vi "Fishing Continuous OCR wit Max Likelihood P Stimuli.vi"() -> ()   [LabVIEW 2019]
doc: "This VI captures the region of the screen and displays it on the front panel continuously.\nCan be used to develop remote desktop applications."
uses:
  System.Drawing
  <vilib>/wsapi/NI_WebServices.lvlib
  <vilib>/Utility/miscctls.llb/LVBoundsTypeDef.ctl
  <vilib>/Utility/inputDevices.llb/closeMouse.vi
  <vilib>/Instr/_visa.llb/VISA Configure Serial Port (Instr).vi
  <vilib>/Utility/inputDevices.llb/mouseAcquire.vi
panel:
  in  "P Trig":bool
  out "P Command":string
  in  "P Stimuli":bool
  out "Length":i32
  out "Array Reset":bool
  out "TXB":bool
  out "Scan Cycle":dbl
  out "read buffer":string
  out "Max Likelihood Output":string
  out "Max Index":i32
  in  "Manual Reset Array":bool
  out "Input Likelihood":dbl[](array[numeric])
  out "Possible Inputs":string[](array[string])
  out "Init Error":errorcluster
  out "Tx":string
  out "Return Count":u32
  out "COM Status":bool
  in  "MC COM Port":refnum<visa-resource-name>="COM5"
  out "Processed Image":T1(plugin-control)
  out "Filtered String Output":string
  in  "Delay (ms)":i32=100
  in  "Error In":errorcluster
  out "Mouse y":dbl
  out "Mouse x":dbl
  in  "Height (px)":i32=100
  in  "Width (px)":i32=600
  out "Screen Capture":picture
  in  "stop":bool
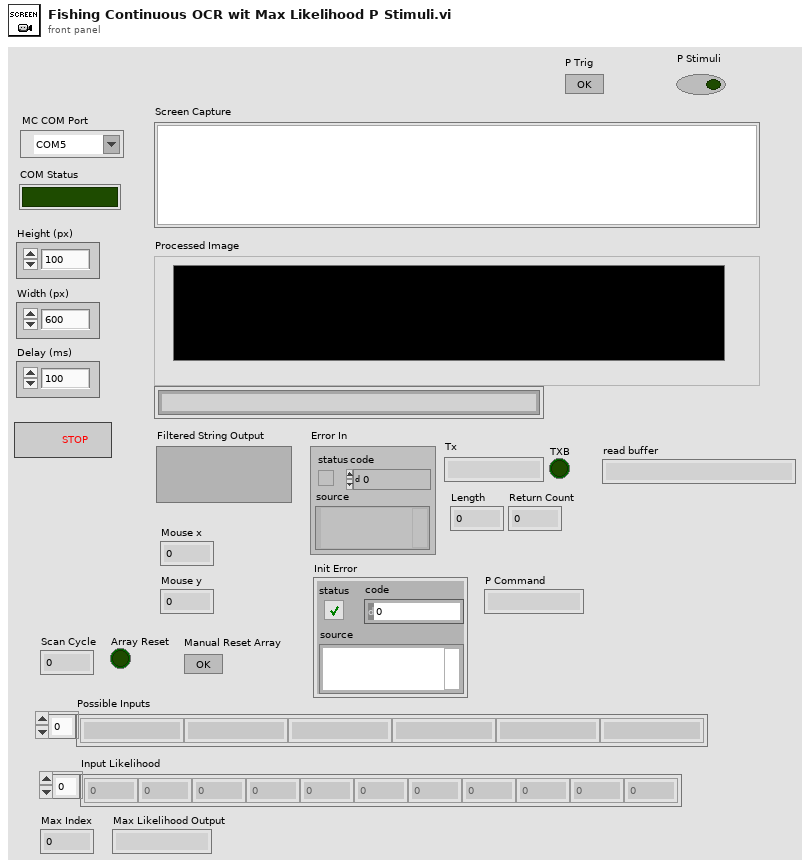
[diagram p1: front panel]
types:
  T1 = typedef "IMAQ Image.ctl" = refnum<image>
  T2 = typedef "LVBoundsTypeDef.ctl" = cluster{"Width":u32, "Height":u32}
  T3 = typedef "Image Type" = u32
  T4 = cluster{"Horizontal":i32, "Vertical":i32, "Scrolling":i32}
  T5 = typedef "imagedata.ctl" = cluster{"image type":i32, "image depth":i32, "image":u8[], "mask":u8[], "colors":u32[], "Rectangle":cluster{"left":i16, "top":i16, "right":i16, "bottom":i16}}
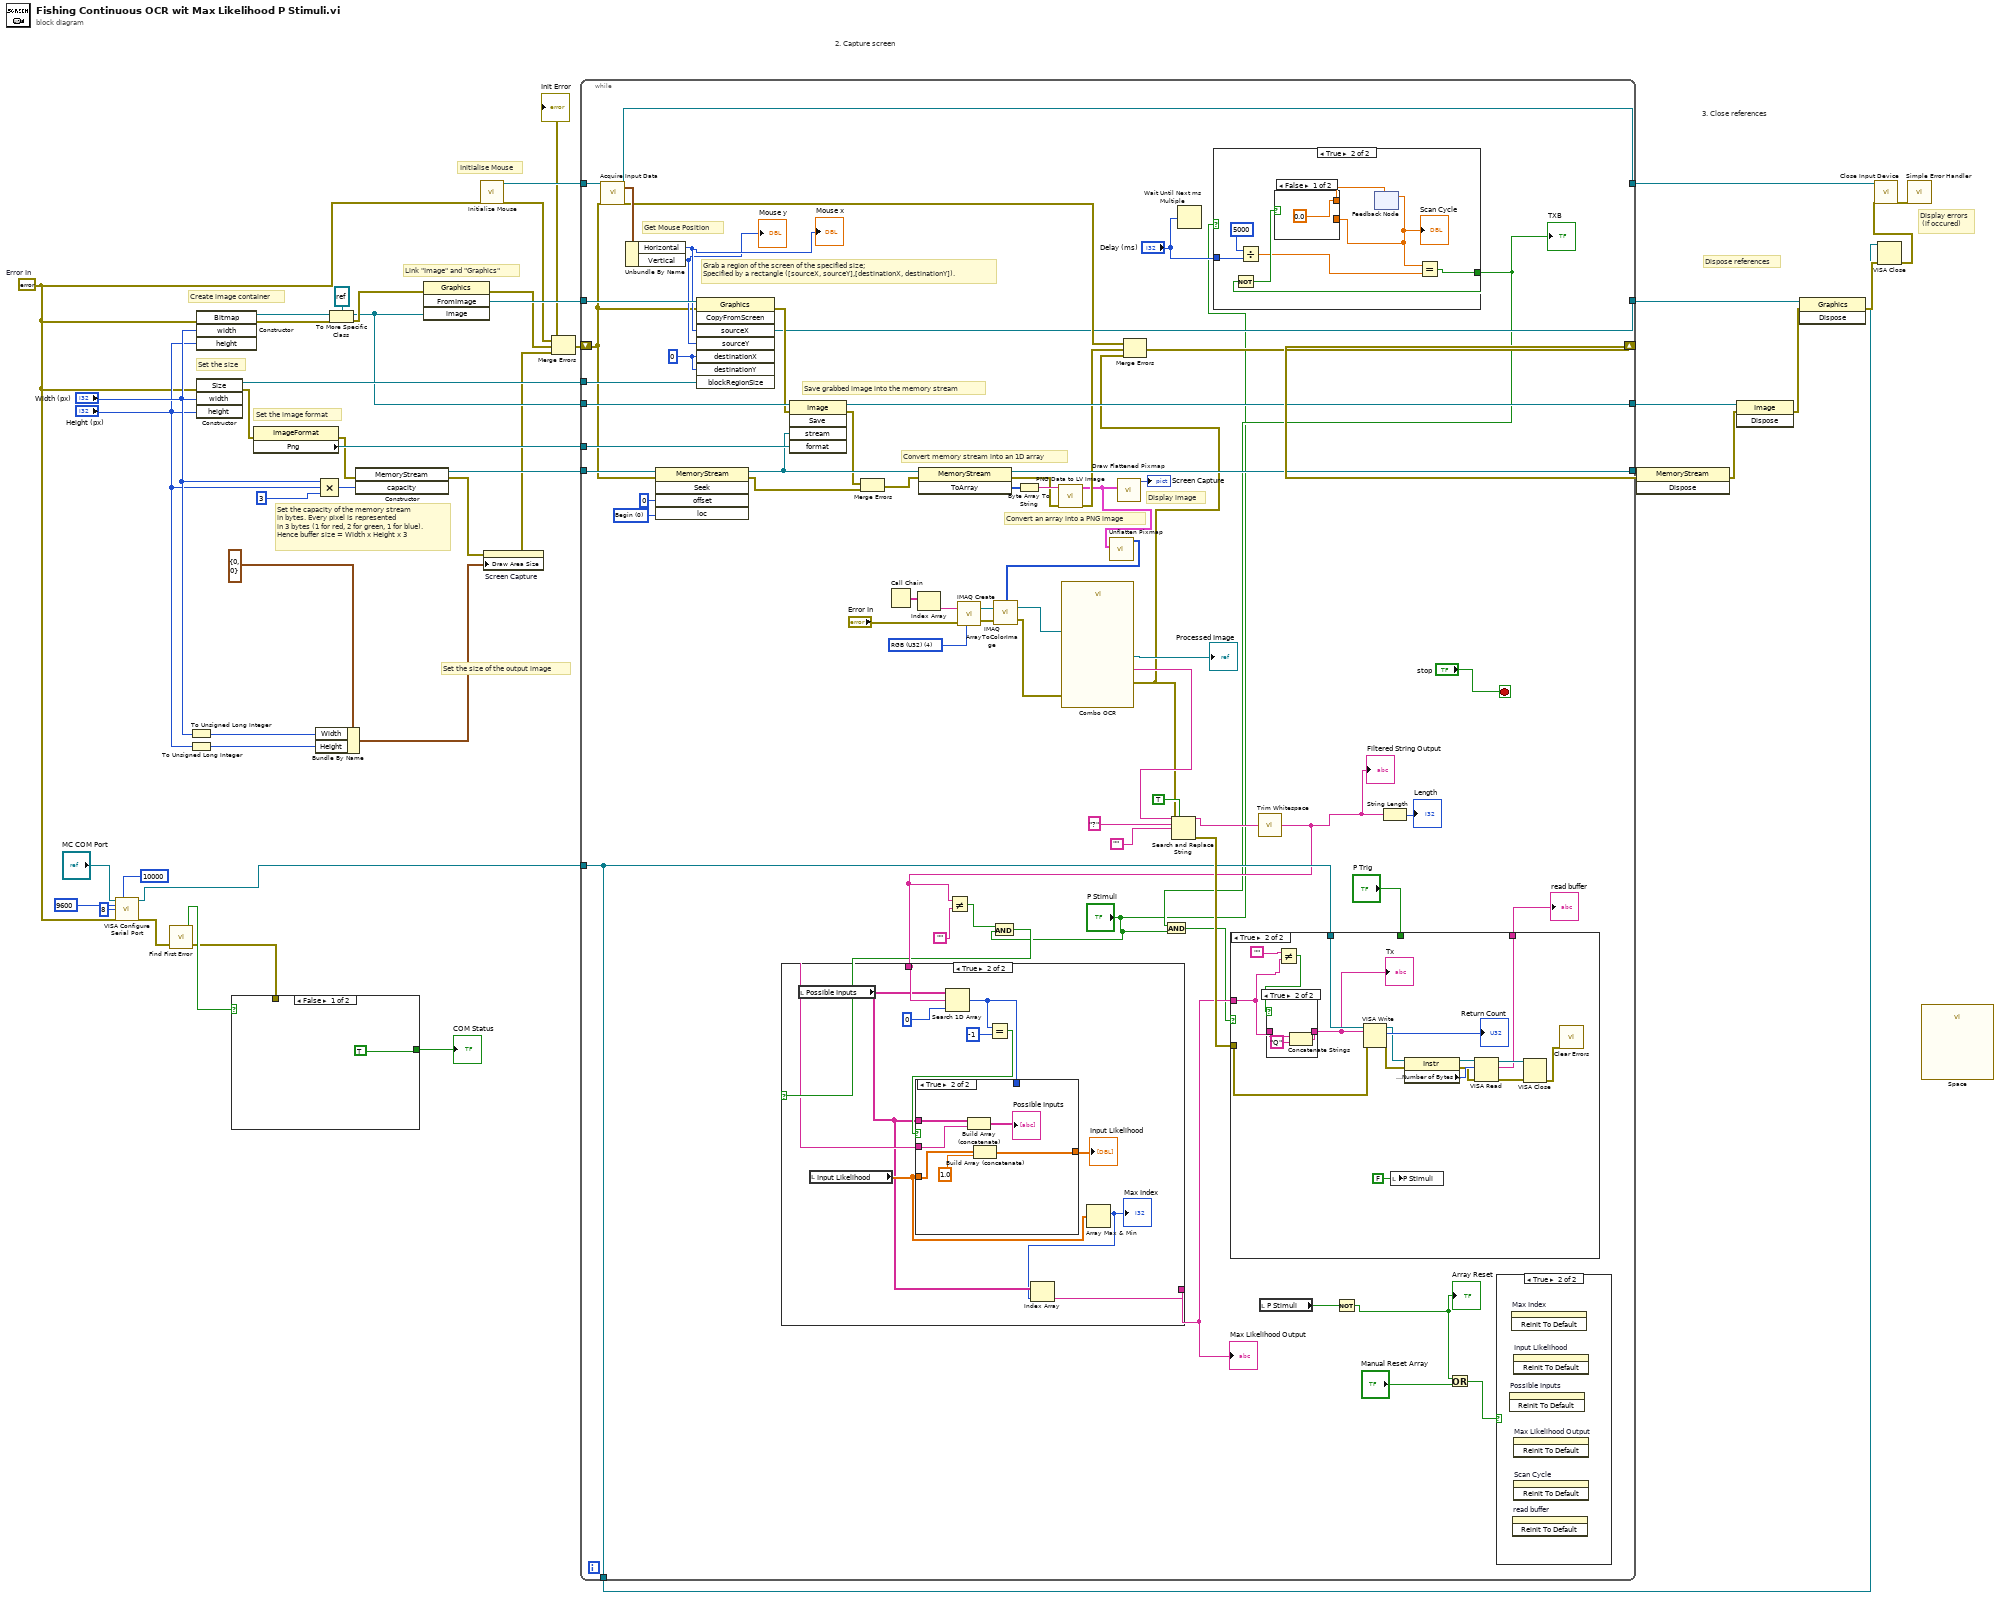
[diagram p0: block diagram]
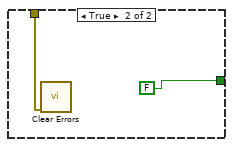
[diagram p2: hidden frame]
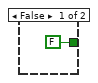
[diagram p3: hidden frame]
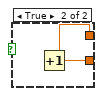
[diagram p4: hidden frame]
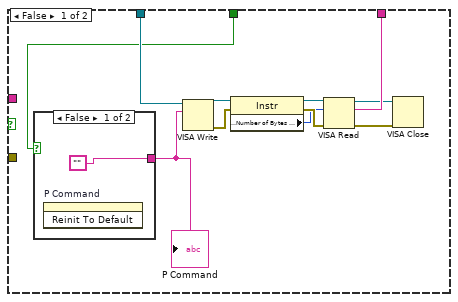
[diagram p5: hidden frame]
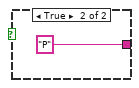
[diagram p6: hidden frame]
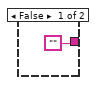
[diagram p7: hidden frame]
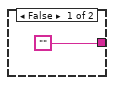
[diagram p8: hidden frame]
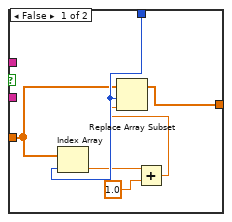
[diagram p9: hidden frame]
diagram:
  w12 = errorcluster {"status"=FALSE, "code"=0, "source"=""}  # Error In
  # "Link \"Image\" and \"Graphics\""
  # "Set the size"
  # "Create image container"
  # "3. Close references"
  # "2. Capture screen"
  # "Display errors\n (if occured)"
  # "Dispose references"
  # "Set the image format"
  # "Set the size of the output image"
  # "Set the capacity of the memory stream\nin bytes. Every pixel is represented\nin 3 bytes (1 for red, 2 for green, 1 for blue).\nHence buffer size = Width x Height x 3"
  # "Initialise Mouse"
  n1 = call-poly "VISA Configure Serial Port"("VISA resource name"="MC COM Port", "timeout (10sec)"=u32 10000, "baud rate (9600)"=u32 9600, "data bits (8)"=u16 8, "error in (no error)"=w12) -> ("VISA resource name out"=w1:refnum<visa-resource-name>, "error out"=w11:errorcluster)  [unwired: 9 in]
  n2 = call <vilib>:"Find First Error.vi"("error in (no error)"=w11) -> ("error out"=w8:errorcluster, "error?"=w10:bool)  [unwired: 3 in]
  n3 = To Unsigned Long Integer(number="Width (px)") -> (unsigned 32bit integer=w20:u32)
  n4 = To Unsigned Long Integer(number="Height (px)") -> (unsigned 32bit integer=w18:u32)
  n5 = constructor class="Bitmap"(error in=w12, "width"="Width (px)", "height"="Height (px)") -> (reference out=w40:refnum<k24>, error out=w43:errorcluster)  [unwired: 2 in, 3 out]
  n6 = constructor class="Size"(error in=w12, "width"="Width (px)", "height"="Height (px)") -> (reference out=w38:refnum<k24>, error out=w29:errorcluster)  [unwired: 2 in, 3 out]
  n7 = case shown="False" w10 {
    tunnel: [TRUE FALSE] -> w9
    tunnel: w8 -> [_ w48]
    frame False {
    }
    frame True {
      n8 = call <vilib>:"Clear Errors.vi"("error in (no error)"=w48) -> ()  [unwired: 5 in, 2 out]
    }
  }
  "COM Status" <- w9
  n9 = property class="ImageFormat"(error in=w29) -> (error out=w28:errorcluster, "Png"=w37:refnum<k24>)  [unwired: 1 in, 1 out]
  n10 = Bundle By Name(cluster=T2 {"Width"=0, "Height"=0} ("Draw Area Size"), "Width"=w20, "Height"=w18) -> (w24:T2)
  n11 = Compound Arithmetic op=MULTIPLY("Width (px)", "Height (px)", 3 ("value")) -> (w32:i32)
  n12 = To More Specific Class(target class=refnum<k24> refnum, reference=w40, error in=w43) -> (specific class reference=w31:refnum<k24>, error out=w44:errorcluster)
  n13 = constructor class="MemoryStream"(error in=w28, "capacity"=w32) -> (reference out=w34:refnum<k24>, error out=w23:errorcluster)  [unwired: 2 in, 2 out]
  n14 = invoke class="Graphics" method="FromImage"(error in=w44, "image"=w31) -> (error out=w27:errorcluster, "FromImage"=w41:refnum<k24>)  [unwired: 2 in, 2 out]
  n15 = call <vilib>:"Initialize Mouse.vi"("error in (no error)"=w12) -> ("error out"=w25:errorcluster, "device ID"=w46:refnum<k1>)  [unwired: 9 in]
  n16 = property on="Screen Capture" class="Pict"(error in=w23, "Draw Area Size"=w24) -> (error out=w22:errorcluster)  [unwired: 1 in, 1 out]
  n17 = Merge Errors(w25, w27, w22) -> (w26:errorcluster)
  "Init Error" <- w26
  n18 = while {
    tunnel: w46 -> [w114]
    tunnel: [w112] -> w45
    tunnel: w41 -> [w111]
    tunnel: [w108] -> w39
    tunnel: w38 -> [w107]
    tunnel: w37 -> [w106]
    tunnel: [w105] -> w36
    tunnel: w34 -> [w104]
    tunnel: w31 -> [w98]
    shift-right: [w90] -> w14
    shift-left: w26 -> [w69]
    tunnel: [w89] -> w17
    tunnel: w1 -> [w61]
    tunnel: [w61] -> w5
    stop <- "stop" stop-if-true
    w81 = T3 4 items=["Grayscale (U8)", "Grayscale (I16)", "Grayscale (SGL)", "Complex (CSG)", "RGB (U32)", "HSL (U32)", "RGB (U64)", "Grayscale (U16)"] ("Image Type")
    w99 = 0 ("destinationX")
    w102 = 0 items=["Begin", "Current", "End"] ("loc")
    # "Display image"
    # "Convert an array into a PNG image"
    # "Convert memory stream into an 1D array"
    # "Save grabbed image into the memory stream"
    # "Grab a region of the screen of the specified size;\nSpecified by a rectangle ([sourceX, sourceY],[destinationX, destinationY])."
    # "Get Mouse Position"
    n19 = call-poly <vilib>:"Acquire Input Data.vi"("device ID"=w114, "error in (no error)"=w69) -> ("device ID"=w112:refnum<k1>, "axis info"=w113:T4, "error out"=w92:errorcluster)  [unwired: 14 in, 1 out]
    n20 = Unbundle By Name(w113) -> ("Horizontal"=w88:i32, "Vertical"=w87:i32)
    "Mouse x" <- w88
    "Mouse y" <- w87
    n21 = invoke class="MemoryStream" method="Seek"(reference=w104, error in=w69, "offset"=i64 0, "loc"=w102) -> (reference out=w100:refnum<k24>, error out=w95:errorcluster)  [unwired: 1 in, 3 out]
    n22 = invoke class="Graphics" method="CopyFromScreen"(reference=w111, error in=w69, "sourceX"=w88, "sourceY"=w87, "destinationX"=w99, "destinationY"=w99, "blockRegionSize"=w107) -> (reference out=w89:refnum<k24>, error out=w93:errorcluster)  [unwired: 1 in, 6 out]
    n23 = invoke class="Image" method="Save"(reference=w98, error in=w93, "stream"=w100, "format"=w106) -> (reference out=w105:refnum<k24>, error out=w96:errorcluster)  [unwired: 1 in, 3 out]
    n24 = Merge Errors(w96, w95) -> (w94:errorcluster)
    n25 = Call Chain() -> (call chain=w83:string[])
    n26 = Index Array(array=w83) -> (element=w84:string)  [unwired: 1 in]
    n27 = invoke class="MemoryStream" method="ToArray"(reference=w100, error in=w94) -> (reference out=w108:refnum<k24>, error out=w97:errorcluster, "ToArray"=w110:u8[])  [unwired: 1 in]
    n28 = call "IMAQ Create"("Image Name"=w84, "Image Type"=w81, "error in (no error)"="Error In") -> ("New Image"=w80:T1, "error out"=w79:errorcluster)  [unwired: 1 in, 1 out]
    n29 = Byte Array To String(unsigned byte array=w110) -> (string=w109:string)
    n30 = call <vilib>:"PNG Data to LV Image.vi"("error in (no error)"=w97, "png data"=w109) -> ("error out"=w91:errorcluster, "image data"=w86:T5)  [unwired: 8 in]
    n31 = call <vilib>:"Unflatten Pixmap.vi"("image data"=w86) -> ("24-bit pixmap"=w85:u32[][])  [unwired: 4 in, 6 out]
    n32 = call "IMAQ ArrayToColorImage"("Image Pixels (U32)"=w85, "Image"=w80, "error in (no error)"=w79) -> ("Image Out"=w77:T1, "error out"=w78:errorcluster)  [unwired: 2 in]
    n33 = call "Combo OCR"("Image In"=w77, "error in"=w78) -> ("Image Out"=→"Processed Image":T1, "String (OCR/OCV 2)"=w73:string, "error out"=w68:errorcluster)  [unwired: 23 in]
    n34 = call <vilib>:"Draw Flattened Pixmap.vi"("image data"=w86) -> ("new picture"=→"Screen Capture":picture)  [unwired: 8 in]
    n35 = Merge Errors(w92, w91, w68) -> (w90:errorcluster)
    n36 = Search and Replace String(replace all?=TRUE ("replace all? (F)"), input string=w73, search string="?", replace string="", error in=w68) -> (result string=w72:string, error out=w67:errorcluster)  [unwired: 3 in, 2 out]
    n37 = Wait Until Next ms Multiple(millisecond multiple="Delay (ms)") -> ()  [unwired: 1 out]
    n38 = case shown="True" "P Stimuli" {
      tunnel: "Delay (ms)" -> [_ w122]
      tunnel: [FALSE w116] -> w55
      frame False {
      }
      frame True {
        n39 = Divide(x=5000, y=w122) -> (x/y=w117:dbl)
        n40 = feedback #1() -> (w119:dbl)  [unwired: 1 in]
        "Scan Cycle" <- w119
        n41 = Equal?(x=w119, y=w117) -> (x = y?=w116:bool)
        n42 = Not(x=w116) -> (.not. x?=w120:bool)
        n43 = case shown="False" w120 {
          tunnel: [0.0 w125] -> w121
          tunnel: w119 -> [_ w124]
          frame False {
          }
          frame True {
            n44 = Increment(x=w124) -> (x+1=w125:dbl)
          }
        }
        n45 = feedback-in #1(w121) -> ()
      }
    }
    "TXB" <- w55
    n46 = And(x=w55, y="P Stimuli") -> (x .and. y?=w58:bool)
    n47 = call <vilib>:"Trim Whitespace.vi"("string"=w72) -> ("trimmed string"=w60:string)  [unwired: 1 in]
    "Filtered String Output" <- w60
    n48 = Not Equal?(x=w60, y="") -> (x != y?=w57:bool)
    n49 = And(x=w57, y="P Stimuli") -> (x .and. y?=w56:bool)
    n50 = case shown="True" w56 {
      tunnel: w60 -> [_ w165]
      tunnel: ["" w161] -> w65
      frame False {
      }
      frame True {
        n51 = local read "Possible Inputs"() -> (w163:string[])
        n52 = local read "Input Likelihood"() -> (w164:dbl[])
        n53 = Search 1D Array(1D array=w163, element=w165, start index (0)=0) -> (index of element=w167:i32)
        n54 = Equal?(x=w167, y=-1) -> (x = y?=w168:bool)
        n55 = case shown="True" w168 {
          tunnel: w163 -> [_ w182]
          tunnel: w165 -> [_ w181]
          tunnel: w167 -> [w176 _]
          tunnel: w164 -> [w172 w178]
          tunnel: [w171 w179] -> w166
          frame False {
            n56 = Index Array(array=w172, index=w176) -> (element=w174:dbl)
            n57 = Add(x=w174, y=1.0) -> (x+y=w173:dbl)
            n58 = Replace Array Subset(array=w172, new element=w173, index=w176) -> (w171:dbl[])
          }
          frame True {
            n59 = Build Array (concatenate)(w182, w181) -> (→"Possible Inputs":string[])
            n60 = Build Array (concatenate)(w178, 1.0 ("new element/subarray")) -> (w179:dbl[])
          }
        }
        "Input Likelihood" <- w166
        n61 = Array Max & Min(array=w164) -> (max index (indices)=w162:i32)  [unwired: 3 out]
        "Max Index" <- w162
        n62 = Index Array(array=w163, index=w162) -> (element=w161:string)
      }
    }
    "Max Likelihood Output" <- w65
    n63 = case shown="True" w58 {
      tunnel: w61 -> [w136 w155]
      tunnel: w67 -> [_ w153]
      tunnel: w65 -> [_ w145]
      tunnel: [w129 w140] -> w51
      tunnel: "P Trig" -> [w128 _]
      frame False {
        n64 = case shown="False" w128 {
          tunnel: ["" "P"] -> w135
          frame False {
            n65 = invoke on="P Command" class="Str" method="Reinit To Default"() -> ()  [unwired: 3 in, 3 out]
          }
          frame True {
          }
        }
        "P Command" <- w135
        n66 = VISA Write(VISA resource name=w136, write buffer=w135) -> (VISA resource name out=w131:refnum<visa-resource-name>, error out=w130:errorcluster)  [unwired: 1 in, 1 out]
        n67 = property class="Instr"(reference=w131, error in=w130) -> (reference out=w132:refnum<visa-resource-name>, error out=w134:errorcluster, "Serial Settings:Number of Bytes at Serial Port"=w133:u32)
        n68 = VISA Read(VISA resource name=w132, byte count=w133, error in (no error)=w134) -> (VISA resource name out=w126:refnum<visa-resource-name>, read buffer=w129:string, error out=w127:errorcluster)  [unwired: 1 out]
        n69 = VISA Close(VISA resource name=w126, error in (no error)=w127) -> ()  [unwired: 1 out]
      }
      frame True {
        n70 = Not Equal?(x="", y=w145) -> (x != y?=w147:bool)
        n71 = case shown="True" w147 {
          tunnel: ["" w159] -> w144
          tunnel: w145 -> [_ w158]
          frame False {
          }
          frame True {
            n72 = Concatenate Strings(w158, "Q" ("string")) -> (w159:string)
          }
        }
        "Tx" <- w144
        n73 = VISA Write(VISA resource name=w155, write buffer=w144, error in (no error)=w153) -> (VISA resource name out=w152:refnum<visa-resource-name>, return count=→"Return Count":u32, error out=w151:errorcluster)
        n74 = local write "P Stimuli"(FALSE ("P Stimuli")) -> ()
        n75 = property class="Instr"(reference=w152, error in=w151) -> (reference out=w150:refnum<visa-resource-name>, error out=w148:errorcluster, "Serial Settings:Number of Bytes at Serial Port"=w149:u32)
        n76 = VISA Read(VISA resource name=w150, byte count=w149, error in (no error)=w148) -> (VISA resource name out=w143:refnum<visa-resource-name>, read buffer=w140:string, error out=w142:errorcluster)  [unwired: 1 out]
        n77 = VISA Close(VISA resource name=w143, error in (no error)=w142) -> (error out=w141:errorcluster)
        n78 = call <vilib>:"Clear Errors.vi"("error in (no error)"=w141) -> ()  [unwired: 5 in, 2 out]
      }
    }
    "read buffer" <- w51
    n79 = local read "P Stimuli"() -> (w53:bool)
    n80 = Not(x=w53) -> (.not. x?=w52:bool)
    "Array Reset" <- w52
    n81 = String Length(string=w60) -> (length=→"Length":i32)
    n82 = Or(x=w52, y="Manual Reset Array") -> (x .or. y?=w64:bool)
    n83 = case shown="True" w64 {
      frame False {
      }
      frame True {
        n84 = invoke on="Possible Inputs" class="Arr (strict)" method="Reinit To Default"() -> ()  [unwired: 3 in, 3 out]
        n85 = invoke on="Max Index" class="DigNum (strict)" method="Reinit To Default"() -> ()  [unwired: 3 in, 3 out]
        n86 = invoke on="read buffer" class="Str" method="Reinit To Default"() -> ()  [unwired: 3 in, 3 out]
        n87 = invoke on="Input Likelihood" class="Arr (strict)" method="Reinit To Default"() -> ()  [unwired: 3 in, 3 out]
        n88 = invoke on="Max Likelihood Output" class="Str" method="Reinit To Default"() -> ()  [unwired: 3 in, 3 out]
        n89 = invoke on="Scan Cycle" class="DigNum (strict)" method="Reinit To Default"() -> ()  [unwired: 3 in, 3 out]
      }
    }
  }
  n90 = invoke class="MemoryStream" method="Dispose"(reference=w39, error in=w14) -> (error out=w35:errorcluster)  [unwired: 1 in, 2 out]
  n91 = invoke class="Image" method="Dispose"(reference=w36, error in=w35) -> (error out=w16:errorcluster)  [unwired: 1 in, 2 out]
  n92 = invoke class="Graphics" method="Dispose"(reference=w17, error in=w16) -> (error out=w7:errorcluster)  [unwired: 1 in, 2 out]
  n93 = VISA Close(VISA resource name=w5, error in (no error)=w7) -> (error out=w6:errorcluster)
  n94 = call-poly <vilib>:"Close Input Device.vi"("error in (no error)"=w6, "device ID"=w45) -> ("error out"=w15:errorcluster)  [unwired: 8 in]
  n95 = call <vilib>:"Simple Error Handler.vi"("error in (no error)"=w15) -> ()  [unwired: 4 in, 5 out]
  n96 = call "Space"() -> ()  [unwired: 24 in, 4 out]
